vi "test_Add Response ByteCount_UseChannel.vi"(8 "error in (no error)":errorcluster, 11 "TestCase in":refnum<class "Instrument Addon Scripting API Messages Unit Tests.lvclass">) -> (0 "error out":errorcluster, 3 "TestCase out":refnum<class "Instrument Addon Scripting API Messages Unit Tests.lvclass">)   [LabVIEW 2018, in "Instrument Addon Scripting API Messages Unit Tests.lvclass"]
uses:
  Instrument Addon Scripting API Messages Unit Tests.lvclass
  Addon/Addon Shared/Types/Response Parameters.ctl
  Addon/Addon Shared/Types/Linked Channel Cluster.ctl
  Addon/Addon Shared/Types/Response Wait Type.ctl
  Addon/Addon Shared/Types/FG Control.ctl
  APIs/Scripting API/TypeDefs/ByteCount Response Settings.ctl
  APIs/Scripting API/TypeDefs/Linked Channel.ctl
  <vilib>/NI Veristand/Custom Device API/Custom Device Item Ref.ctl
  Addon/Addon Shared/SubVIs/Constants.vi
  <vilib>/NI/NI VeriStand Advanced SysDef API/_SubVIs/SysDef.Search.GUID.vi
  <vilib>/NI Veristand/Custom Device API/NI VeriStand - Get Item Property.vi
  <vilib>/NI Veristand/Custom Device API/Get Item Property (String).vi
  <vilib>/NI Veristand/Custom Device API/Get Item Property (String Array).vi
  <vilib>/NI Veristand/Custom Device API/Get Item Property (Double).vi
  <vilib>/NI Veristand/Custom Device API/Get Item Property (U32).vi
  <vilib>/NI Veristand/Custom Device API/Get Item Property (Boolean).vi
  <vilib>/NI Veristand/Custom Device API/NI VeriStand - Set Item Property.vi
  <vilib>/NI Veristand/Custom Device API/Set Item Property (String).vi
  <vilib>/NI Veristand/Custom Device API/Set Item Property (String Array).vi
  <vilib>/NI Veristand/Custom Device API/Set Item Property (Double).vi
  <vilib>/NI Veristand/Custom Device API/Set Item Property (U32).vi
  <vilib>/NI Veristand/Custom Device API/Set Item Property (Boolean).vi
  APIs/Scripting API/Messages/Add Response - Byte Count.vi
  <vilib>/addons/_JKI Toolkits/VI Tester/TestCase.llb/TestCase.lvclass
  Instrument Addon Scripting API Test Assets/Instrument Addon Scripting API Test Assets.lvclass
  APIs/Scripting API/Instrument Addon Scripting API.lvlib
  <vilib>/NI Veristand/Custom Device API/Custom Device API.lvlib
  Addon/Addon Shared/Instrument Addon Shared.lvlib
  <vilib>/NI/NI VeriStand Advanced SysDef API/SysDef API/Advanced System Definition.lvlib
  C:/Program Files (x86)/National Instruments/LabVIEW 2018/vi.lib/addons/_JKI Toolkits/VI Tester/TestCase.llb/TestCase.lvclass
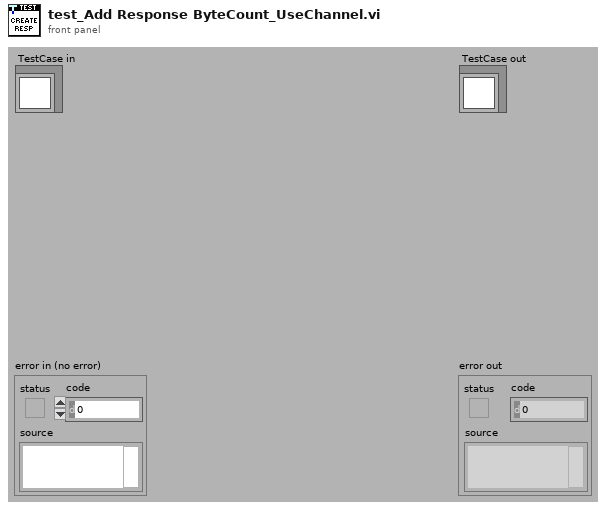
[diagram p1: front panel]
types:
  T1 = typedef "Instrument Addon Scripting API.lvlib/ByteCount Response Settings.ctl" = cluster{"Response Format":string, "Linked Channels":T2[], "Byte Count":i32, "Use Byte Count channel":bool, "Channel Refnum":T3}
  T2 = typedef "Instrument Addon Scripting API.lvlib/Linked Channel.ctl" = cluster{"Variable Name":string, "Channel Refnum":T3}
  T3 = typedef "Custom Device API.lvlib/Custom Device Item Ref.ctl" = u64
  T4 = typedef "Instrument Addon Shared.lvlib/FG Control.ctl" = enum16{"Get", "Set"}
  T5 = typedef "Instrument Addon Shared.lvlib/Response Parameters.ctl" = cluster{"Response":string, "Linked Channels":T6[], "Type Value":dbl, "Wait Type":T7, "Use Channel":bool, "Channel Path":string}
  T6 = typedef "Instrument Addon Shared.lvlib/Linked Channel Cluster.ctl" = cluster{"Variable Name":string, "GUID":string}
  T7 = typedef "Instrument Addon Shared.lvlib/Response Wait Type.ctl" = enum16{"Byte Count", "Wait sec"}
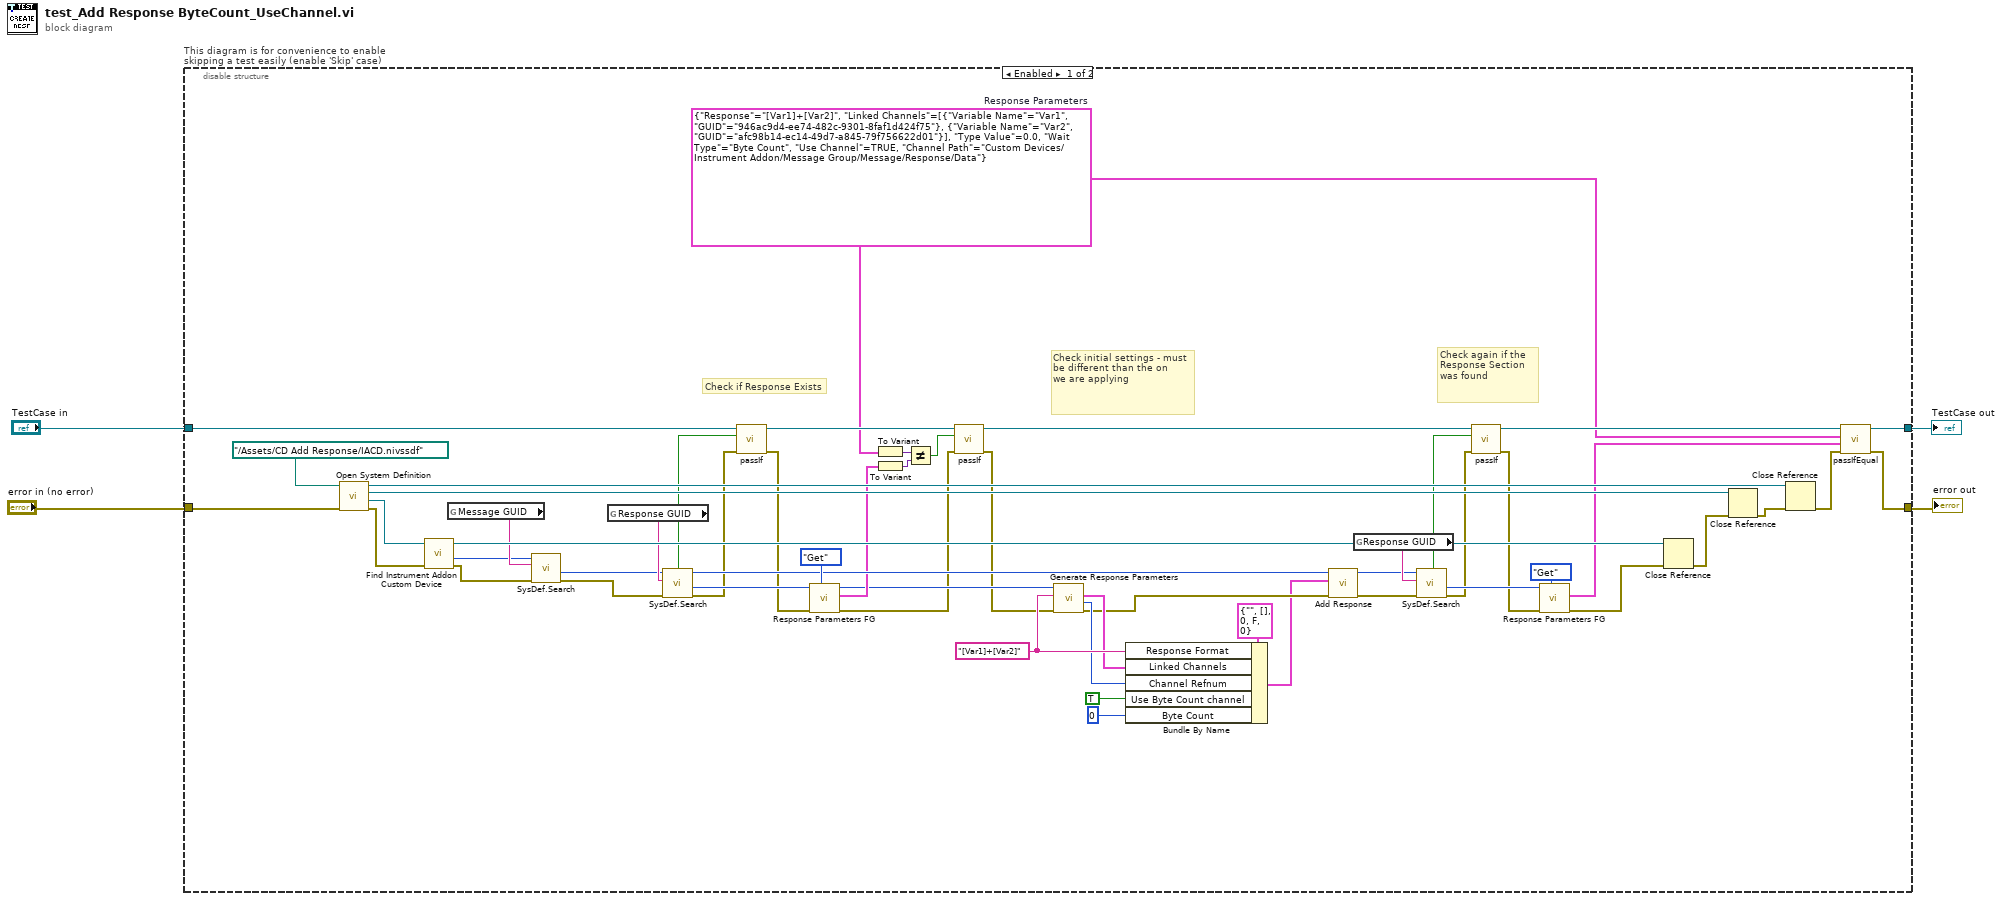
[diagram p0: block diagram]
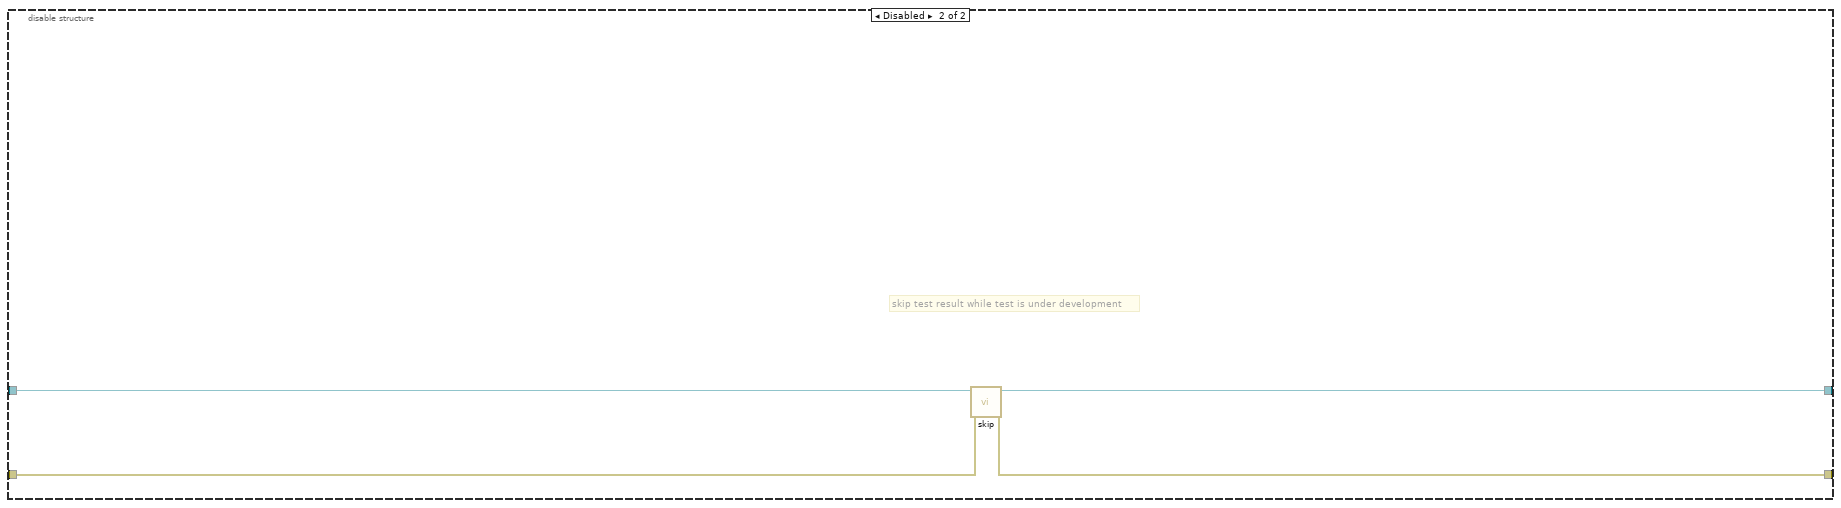
[diagram p2: hidden frame]
diagram:
  n1 = disable-structure "This diagram is for convenience to enable skipping a test easily (enable 'Skip' case)" shown="Enabled" {
    disable-tunnel: "TestCase in" -> [w31 w62]
    disable-tunnel: [w42 w60] -> w1
    disable-tunnel: [w41 w61] -> w3
    disable-tunnel: "error in (no error)" -> [w57 w59]
    frame Enabled {
      w14 = "[Var1]+[Var2]" ("Response Format")
      w16 = T5 {"Response"="[Var1]+[Var2]", "Linked Channels"=[{"Variable Name"="Var1", "GUID"="946ac9d4-ee74-482c-9301-8faf1d424f75"}, {"Variable Name"="Var2", "GUID"="afc98b14-ec14-49d7-a845-79f756622d01"}], "Type Value"=0.0, "Wait Type"=enum."Byte Count", "Use Channel"=TRUE, "Channel Path"="Custom Devices/Instrument Addon/Message Group/Message/Response/Data"}  # Response Parameters
      # "Check again if the Response Section was found"
      # "Check initial settings - must be different than the on\nwe are applying"
      # "Check if Response Exists"
      n2 = call "Open System Definition.vi"("error in (no error)"=w57, "System Definition File"=path "../Assets/CD Add Response/IACD.nivssdf" ("SDF file")) -> ("error out"=w55:errorcluster, "Target Refnum"=w54:refnum<k24>, "Root Refnum"=w53:refnum<k24>, "System Definition Refnum"=w45:refnum<k24>)  [unwired: 6 in]
      n3 = call "Find Instrument Addon Custom Device.vi"("error in"=w55, "target in"=w54) -> ("error out"=w21:errorcluster, "NodeID"=w18:u64, "target out"=w52:refnum<k24>)  [unwired: 7 in]
      n4 = global read "Constants.vi" "Message GUID"() -> (w19:string)
      n5 = call-poly <vilib>:"SysDef.Search.vi"("error in (no error)"=w21, "GUID"=w19, "nodeID"=w18) -> ("error out"=w20:errorcluster, "Value out"=w17:u64)  [unwired: 5 in, 2 out]
      n6 = global read "Constants.vi" "Response GUID"() -> (w38:string)
      n7 = call-poly <vilib>:"SysDef.Search.vi"("error in (no error)"=w20, "GUID"=w38, "nodeID"=w17) -> ("error out"=w29:errorcluster, "Value out"=w39:u64, "nodeID out"=w37:u64, "Found?"=w30:bool)  [unwired: 5 in]
      n8 = call-dynamic "passIf.vi"("error in (no error)"=w29, "pass"=w30, "TestCase in"=w31) -> ("error out"=w28:errorcluster, "TestCase out"=w27:refnum<class "Instrument Addon Scripting API Messages Unit Tests.lvclass">)  [unwired: 7 in]
      n9 = call "Response Parameters FG.vi"("Action"=FG_Control."Get", "error in (no error)"=w28, "Item Ref in"=w39) -> ("error out"=w8:errorcluster, "Response Parameters"=w36:T5, "Item Ref out"=w9:T3)  [unwired: 6 in]
      n10 = To Variant(anything=w16) -> (Variant=w35:variant)
      n11 = To Variant(anything=w36) -> (Variant=w34:variant)
      n12 = Not Equal?(x=w35, y=w34) -> (x != y?=w33:bool)
      n13 = call-dynamic "passIf.vi"("error in (no error)"=w8, "pass"=w33, "TestCase in"=w27) -> ("error out"=w7:errorcluster, "TestCase out"=w26:refnum<class "Instrument Addon Scripting API Messages Unit Tests.lvclass">)  [unwired: 7 in]
      n14 = call "Generate Response Parameters.vi"("Error In"=w7, "Response String"=w14, "Response Channel in"=w9) -> ("Error Out"=w6:errorcluster, "Wait Channel Ref out"=w12:T3, "Linked Channels"=w13:T2[])  [unwired: 5 in, 1 out]
      n15 = Bundle By Name(cluster=T1 {"Response Format"="", "Linked Channels"=[], "Byte Count"=0, "Use Byte Count channel"=FALSE, "Channel Refnum"=0} ("Settings"), "Response Format"=w14, "Linked Channels"=w13, "Channel Refnum"=w12, "Use Byte Count channel"=TRUE, "Byte Count"=0) -> (w5:T1)
      n16 = call-poly "Add Response.vi"("error in (no error)"=w6, "Settings"=w5, "Message in"=w37) -> ("error out"=w48:errorcluster, "Message out"=w47:T3)  [unwired: 7 in]
      n17 = global read "Constants.vi" "Response GUID"() -> (w49:string)
      n18 = call-poly <vilib>:"SysDef.Search.vi"("error in (no error)"=w48, "GUID"=w49, "nodeID"=w47) -> ("error out"=w25:errorcluster, "Value out"=w46:u64, "Found?"=w24:bool)  [unwired: 5 in, 1 out]
      n19 = call-dynamic "passIf.vi"("error in (no error)"=w25, "pass"=w24, "TestCase in"=w26) -> ("error out"=w23:errorcluster, "TestCase out"=w22:refnum<class "Instrument Addon Scripting API Messages Unit Tests.lvclass">)  [unwired: 7 in]
      n20 = call "Response Parameters FG.vi"("Action"=FG_Control."Get", "error in (no error)"=w23, "Item Ref in"=w46) -> ("error out"=w50:errorcluster, "Response Parameters"=w32:T5)  [unwired: 6 in, 1 out]
      n21 = Close Reference(reference=w52, error in (no error)=w50) -> (error out=w56:errorcluster)
      n22 = Close Reference(reference=w53, error in (no error)=w56) -> (error out=w44:errorcluster)
      n23 = Close Reference(reference=w45, error in (no error)=w44) -> (error out=w43:errorcluster)
      n24 = call-dynamic "passIfEqual.vi"("error in (no error)"=w43, "y"=w32, "x"=w16, "TestCase in"=w22) -> ("error out"=w41:errorcluster, "TestCase out"=w42:refnum<class "Instrument Addon Scripting API Messages Unit Tests.lvclass">)  [unwired: 6 in]
    }
    frame Disabled {
      # "skip test result while test is under development"
      n25 = call <vilib>:"skip.vi"("error in (no error)"=w59, "TestCase in"=w62) -> ("error out"=w61:errorcluster, "TestCase out"=w60:refnum<class "Instrument Addon Scripting API Messages Unit Tests.lvclass">)  [unwired: 8 in]
    }
  }
  "error out" <- w3
  "TestCase out" <- w1
